vi "Complete Multipart Upload.vi"(8 "error in (no error)":errorcluster, 11 "Multipart Upload":refnum<class "Multipart Upload.lvclass">) -> (0 "error out":errorcluster, 1 "ETag":string, 2 "Location":string, 3 "Bucket":refnum<class "Bucket.lvclass">, 4 "Version ID":string)   [LabVIEW 2015, in "NI_AWS_S3.lvlib" / "Multipart Upload.lvclass"]
uses:
  Multipart Upload.lvclass
  Bucket/Bucket.lvclass
  Core/HTTP Request/Name Value Pair.ctl
  Core/HTTP Request/Request Options.ctl
  Core/HTTP Request/Region handling.ctl
  Core/HTTP Request/URL formatting.ctl
  Multipart Upload.lvclass/Multipart Upload.ctl
  Bucket/Bucket.lvclass/Bucket.ctl
  Read Bucket.vi
  Read Parts.vi
  Read Upload ID.vi
  Read Object Key.vi
  Bucket/Read Name.vi
  Core/HTTP Request/HTTP Request.lvclass
  XML Parsing/NI_XML Parsing.lvlib
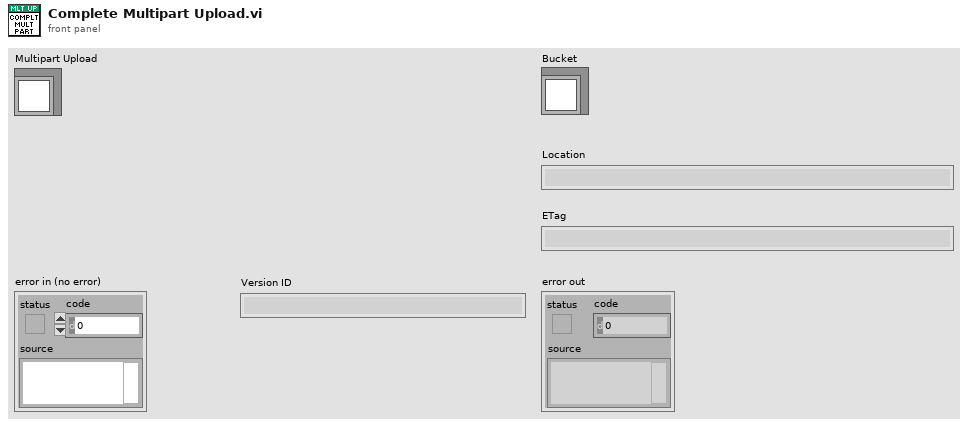
[diagram p1: front panel]
types:
  T1 = typedef "NI_AWS_Core.lvlib/HTTP Request.lvclass/Name Value Pair.ctl" = cluster{"name":string, "value":string}
  T2 = typedef "NI_AWS_Core.lvlib/HTTP Request.lvclass/Region handling.ctl" = enum16{"use region everywhere", "use region (authentication only)", "use region (URL only)", "ignore region everwhere"}
  T3 = typedef "NI_AWS_Core.lvlib/HTTP Request.lvclass/Request Options.ctl" = cluster{"request headers":T1[], "request parameters":T1[], "request body":string, "region handling":T2, "URL formatting":T4}
  T4 = typedef "NI_AWS_Core.lvlib/HTTP Request.lvclass/URL formatting.ctl" = enum16{"region-", "region."}
  T5 = typedef "NI_AWS_S3.lvlib/Part.ctl" = cluster{"Part Number":i32, "Last Modified":timestamp, "ETag":string, "Size":i32}
  T6 = typedef "NI_AWS_Core.lvlib/HTTP Request.lvclass/Response.ctl" = cluster{"Headers":string, "Body":string}
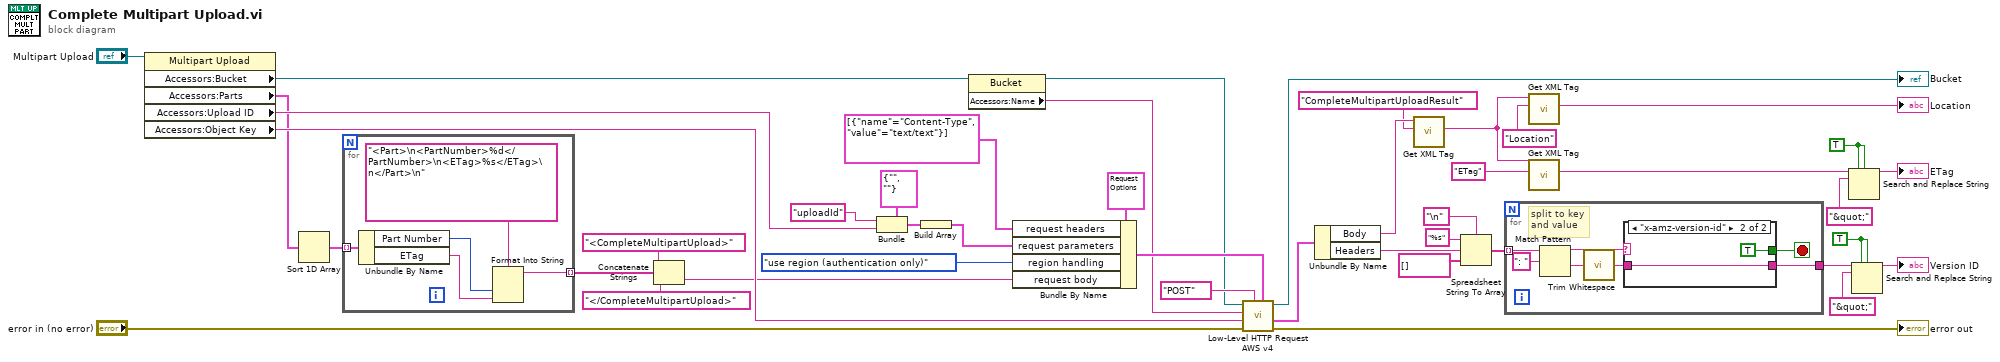
[diagram p0: block diagram]
diagram:
  w2 = TRUE ("replace all? (F)")
  w7 = TRUE ("replace all? (F)")
  n1 = property class="Multipart Upload"(reference="Multipart Upload") -> ("Accessors:Bucket"=w35:refnum<class "Bucket.lvclass">, "Accessors:Parts"=w25:T5[], "Accessors:Upload ID"=w29:string, "Accessors:Object Key"=w32:string)  [unwired: 1 in, 2 out]
  n2 = Sort 1D Array(array=w25) -> (sorted array=w26:T5[])
  n3 = for {
    tunnel: w26 -> [w49] mode=indexing
    tunnel: [w45] -> w27 mode=indexing
    n4 = Unbundle By Name(w49) -> ("Part Number"=w47:i32, "ETag"=w46:string)
    n5 = Format Into String(format string="<Part>\n<PartNumber>%d</PartNumber>\n<ETag>%s</ETag>\n</Part>\n", w47, w46) -> (resulting string=w45:string)  [unwired: 2 in, 1 out]
  }
  n6 = Concatenate Strings("<CompleteMultipartUpload>", w27, "</CompleteMultipartUpload>") -> (w22:string)
  n7 = Bundle(cluster=T1 {"name"="", "value"=""} ("Name Value Pair"), "name"="uploadId" ("format string"), "value"=w29) -> (w43:T1)
  n8 = Build Array(w43) -> (w30:T1[])
  n9 = property class="Bucket"(reference=w35) -> (reference out=w34:refnum<class "Bucket.lvclass">, "Accessors:Name"=w33:string)  [unwired: 1 in, 1 out]
  n10 = Bundle By Name(cluster=T3 {"request headers"=[], "request parameters"=[], "request body"="", "region handling"=enum."use region everywhere", "URL formatting"=enum."region."} ("Request Options"), "request headers"=T1[] [{"name"="Content-Type", "value"="text/text"}], "request parameters"=w30, "region handling"=Region_handling."use region (authentication only)", "request body"=w22) -> (w39:T3)
  n11 = call "Low-Level HTTP Request AWS v4.vi"("Request Options"=w39, "HTTP-Verb"="POST", "error in (no error)"="error in (no error)", "URL Suffix"=w32, "URL Prefix"=w33, "AWS Core in"=w34) -> ("error out"=→"error out":errorcluster, "Response"=w28:T6, "AWS Core out"=→"Bucket":refnum<class "Bucket.lvclass">)  [unwired: 2 in, 1 out]
  n12 = Unbundle By Name(w28) -> ("Body"=w15:string, "Headers"=w16:string)
  n13 = call "Get XML Tag.vi"("Tag name"="CompleteMultipartUploadResult", "XML String in"=w15) -> ("Tag value"=w11:string)  [unwired: 5 in, 4 out]
  n14 = Spreadsheet String To Array(delimiter (Tab)="\n", format string="%s", spreadsheet string=w16, array type (2D Dbl)=string[] []) -> (array=w18:string[])
  n15 = for {
    tunnel: w18 -> [w56] mode=indexing
    tunnel: [w50] -> w9
    stop <- w51 stop-if-true
    # "split to key\nand value"
    n16 = Match Pattern(string=w56, regular expression=": ") -> (before substring=w54:string, after substring=w53:string)  [unwired: 1 in, 2 out]
    n17 = call <vilib>:"Trim Whitespace.vi"("string"=w53) -> ("trimmed string"=w52:string)  [unwired: 1 in]
    n18 = case shown="\"x-amz-version-id\"" w54 {
      tunnel: w52 -> [_ w58]
      tunnel: [_ w58] -> w50
      tunnel: [_ TRUE] -> w51
      frame Default {
      }
      frame "x-amz-version-id" {
      }
    }
  }
  n19 = call "Get XML Tag.vi"("Tag name"="Location", "XML String in"=w11) -> ("Tag value"=→"Location":string)  [unwired: 5 in, 4 out]
  n20 = call "Get XML Tag.vi"("Tag name"="ETag", "XML String in"=w11) -> ("Tag value"=w4:string)  [unwired: 5 in, 4 out]
  n21 = Search and Replace String(replace all?=w2, case sensitive?=w2, input string=w4, search string="&quot;") -> (result string=→"ETag":string)  [unwired: 4 in, 3 out]
  n22 = Search and Replace String(replace all?=w7, case sensitive?=w7, input string=w9, search string="&quot;") -> (result string=→"Version ID":string)  [unwired: 4 in, 3 out]
